vi "Periodic Tasks.vi"(8 "error in":errorcluster) -> ()   [LabVIEW 2018]
doc: "This VI runs in parallel to other tasks. It can contain as many user-defined periodic loops as you need. These can carry out PID or other sorts of timed response."
uses:
  <vilib>/Rock Robotics/WPI/ThirdParty/Phoenix-LabVIEW/Pigeon IMU/CTRE_PigeonIMU_CalibrationMode.ctl
  <vilib>/Rock Robotics/WPI/ThirdParty/Phoenix-LabVIEW/Pigeon IMU/CTRE_PigeonIMU_PigeonState.ctl
  DriveLoopEnum.ctl
  <vilib>/Rock Robotics/WPI/Utilities/WPI_GetSetVariantRefNum.vi
  <vilib>/Rock Robotics/WPI/ThirdParty/Phoenix-LabVIEW/Pigeon IMU/CTRE_PigeonIMU_GetTempStateUpTime.vi
  <vilib>/Rock Robotics/WPI/ThirdParty/Phoenix-LabVIEW/Pigeon IMU/CTRE_PigeonIMU_GetFusedHeading.vi
  <vilib>/Rock Robotics/WPI/ThirdParty/Phoenix-LabVIEW/Motor Controller/Get/CTRE_Phoenix_MotorController_GetVoltage.vi
  <vilib>/Rock Robotics/WPI/ThirdParty/Phoenix-LabVIEW/Motor Controller/Get/CTRE_Phoenix_MotorController_GetSelectedSensorData.vi
  <vilib>/Rock Robotics/WPI/ThirdParty/Phoenix-LabVIEW/Motor Controller/Get/CTRE_Phoenix_MotorController_GetClosedLoopData.vi
panel:
  out "Integral Accumulator":dbl
  out "Percent Power":T1(graph)
  out "Velocity":T2(graph)
  out "Error":cluster{"Closed-loop Error":i32, dbl, dbl}(graph)
  in  "D":dbl
  in  "I":dbl
  in  "P":dbl=1.0
  in  "Percent Max Speed":dbl=0.4
  in  "LowMaxSpeed":i32=7000
  out "Temp/State/UpTime":T5={"CurrentMode"=0, "LastCalError"=0, "CalBooting?"=FALSE, "PigeonState"=enum."Ready", "UpTime"=255, "Temp. (C)"=34.76953125, "Temp Compensation Event Count"=0, "No Motion Event Count"=0} {"CurrentMode" items=["BootTareGryoAccel"=0, "Temperature"=1, "Magnetometer12Pt"=2, "Magnetometer360"=3, "Accelerometer"=5]}
  out "Fused Heading":T6={"Heading"=373.0078125, "Valid?"=FALSE, "Fusing?"=FALSE}
  out "Right Position (Raw Sensor Units)":i32=1024961
  out "Left Position (Raw Sensor Units)":i32=868111
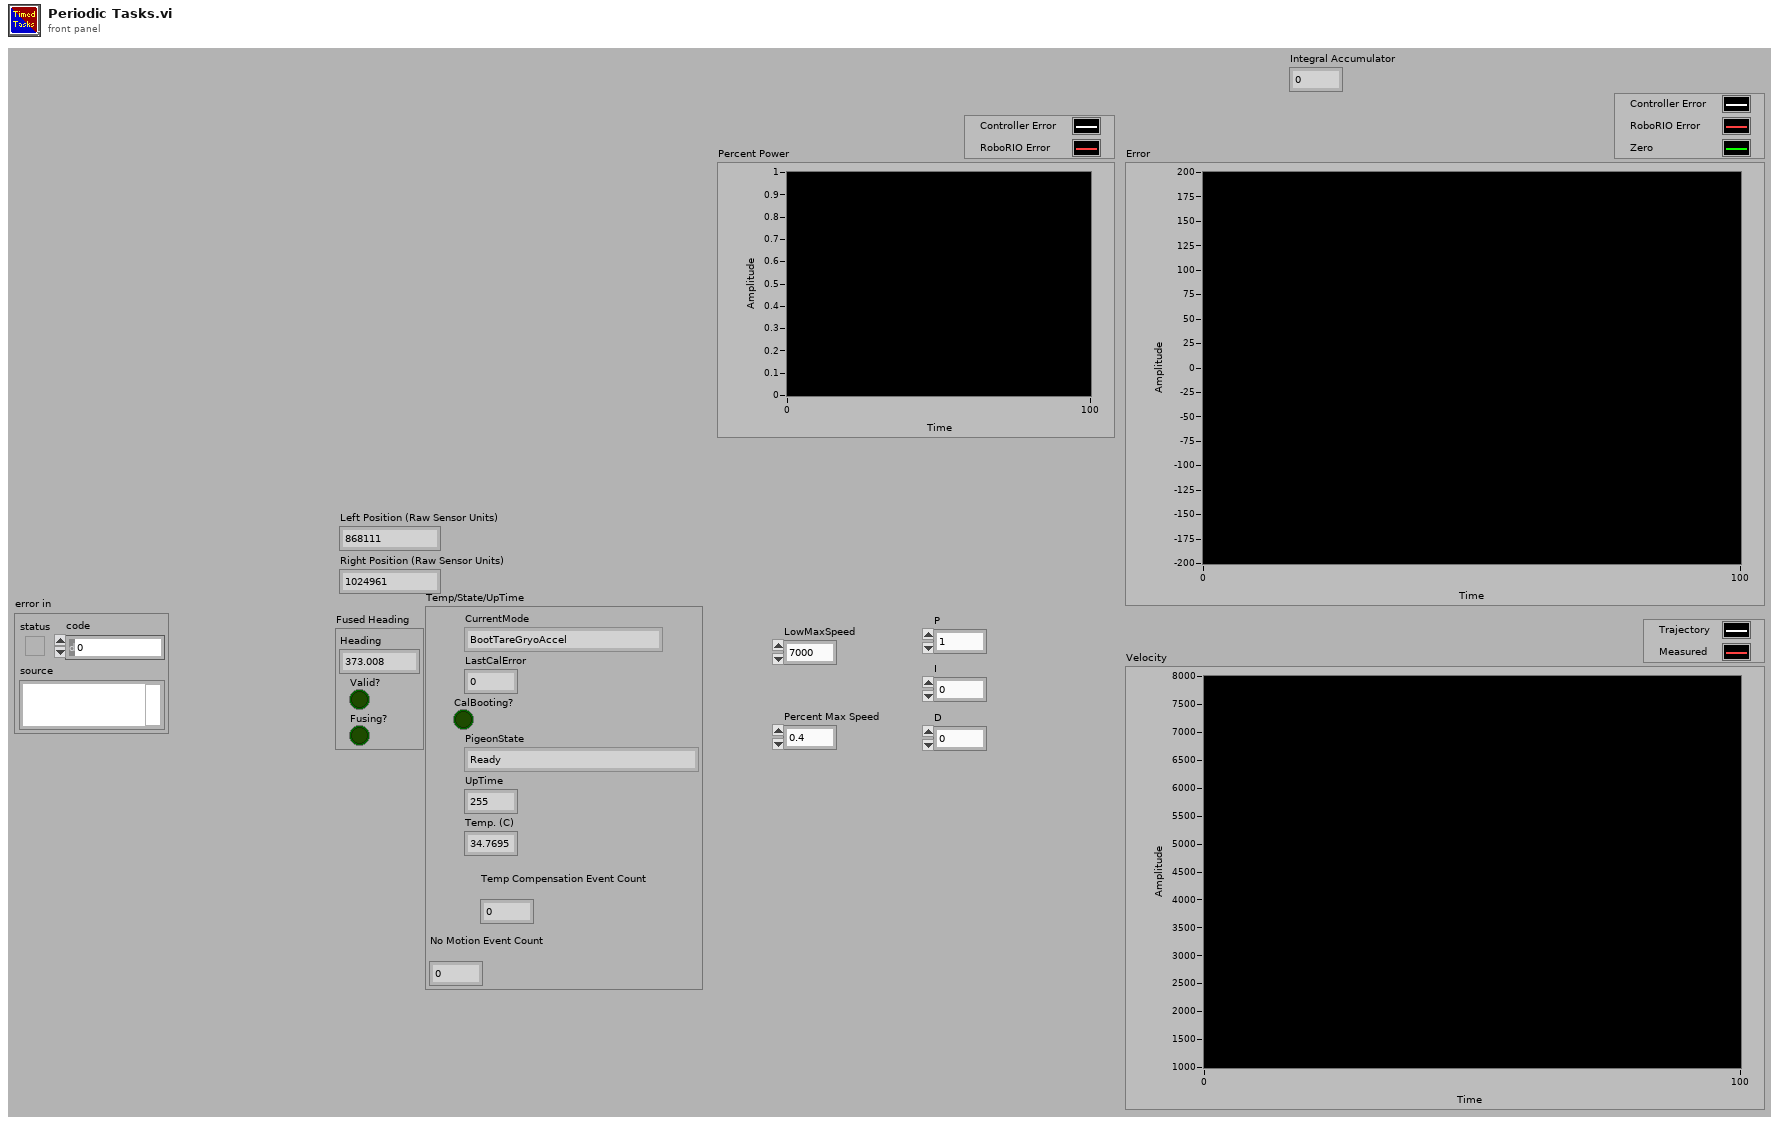
[diagram p1: front panel]
types:
  T1 = cluster{"Percent Output":dbl, "Percent Output":dbl}
  T2 = cluster{"Closed-loop Target":dbl, "Velocity (Raw Sensor Units per 100 ms)":i32}
  T3 = typedef "CTRE_PigeonIMU_CalibrationMode.ctl" = u16
  T4 = typedef "CTRE_PigeonIMU_PigeonState.ctl" = enum16{"NoComm", "Initializing", "Ready", "UserCalibration"}
  T5 = cluster{"CurrentMode":T3, "LastCalError":i32, "CalBooting?":bool, "PigeonState":T4, "UpTime":u32, "Temp. (C)":dbl, "Temp Compensation Event Count":u32, "No Motion Event Count":u32}
  T6 = cluster{"Heading":dbl, "Valid?":bool, "Fusing?":bool}
  T7 = typedef "CTRE_PigeonIMU_DeviceRef.ctl" = cluster{"DeviceStatus":errorcluster, "Device Number":u8, "Type":T8, "Device ID":u32, "Handle":u64, "UsageFrame":u32, "Library Path":path}
  T8 = typedef "CTRE_PigeonIMU_ConnectionType.ctl" = u32
  T9 = typedef "WPI_MotorControlDeviceRef.ctl" = cluster{"DeviceStatus":errorcluster, "Type":T10, "PWM":cluster{"PWM Channel":T11, "DeadBand":T12}, "CAN":cluster{"Device Number":u8, "SetOutput VI Ref":variant, "GetOutput VI Ref":variant, "Enable VI Ref":variant, "Disable VI Ref":variant, "Data":variant}, "Invert":bool, "DIO PWM":cluster{"PWM \"Enable\" Channel":T11, "DIOChannel":T13, "PWM Rate":dbl}}
  T10 = typedef "WPI_MotorControlType.ctl" = enum16{"PWM", "CAN", "DIO PWM"}
  T11 = typedef "FPGA_DIOPWMChannel.ctl" = enum8{"PWM 0", "PWM 1", "PWM 2", "PWM 3", "PWM 4", "PWM 5", "PWM 6", "PWM 7", "PWM 8", "PWM 9", "PWM MXP 0", "PWM MXP 1", "PWM MXP 2", "PWM MXP 3", "PWM MXP 4", "PWM MXP 5", "PWM MXP 6", "PWM MXP 7", "PWM MXP 8", "PWM MXP 9", "Invalid"}
  T12 = typedef "WPI_PWMDeadband.ctl" = cluster{"Name":string, "maxPositivePwm":i32, "minPositivePwm":i32, "centerPwm":i32, "maxNegativePwm":i32, "minNegativePwm":i32, "angularRange":u16}
  T13 = typedef "FPGA_DIOChannel.ctl" = enum8{"DIO 0", "DIO 1", "DIO 2", "DIO 3", "DIO 4", "DIO 5", "DIO 6", "DIO 7", "DIO 8", "DIO 9", "DIO MXP 0", "DIO MXP 1", "DIO MXP 2", "DIO MXP 3", "DIO MXP 4", "DIO MXP 5", "DIO MXP 6", "DIO MXP 7", "DIO MXP 8", "DIO MXP 9", "DIO MXP 10", "DIO MXP 11", "DIO MXP 12", "DIO MXP 13", "DIO MXP 14", "DIO MXP 15", "SPI Port CS1", "SPI Port CS2", "SPI Port CS3", "SPI Port MISO", "SPI Port MOSI", "Invalid"}
  T14 = typedef "WPI_JoystickDevRef.ctl" = cluster{"Device":T15}
  T15 = typedef "WPI_JoystickDeviceEnum.ctl" = enum16{"USB 0", "USB 1", "USB 2", "USB 3", "USB 4", "USB 5"}
  T16 = typedef "DriveLoopEnum.ctl" = enum16{"Manual", "Velocity Control", "Motion Magic"}
  T17 = cluster{dbl, "Velocity (Raw Sensor Units per 100 ms)":i32}
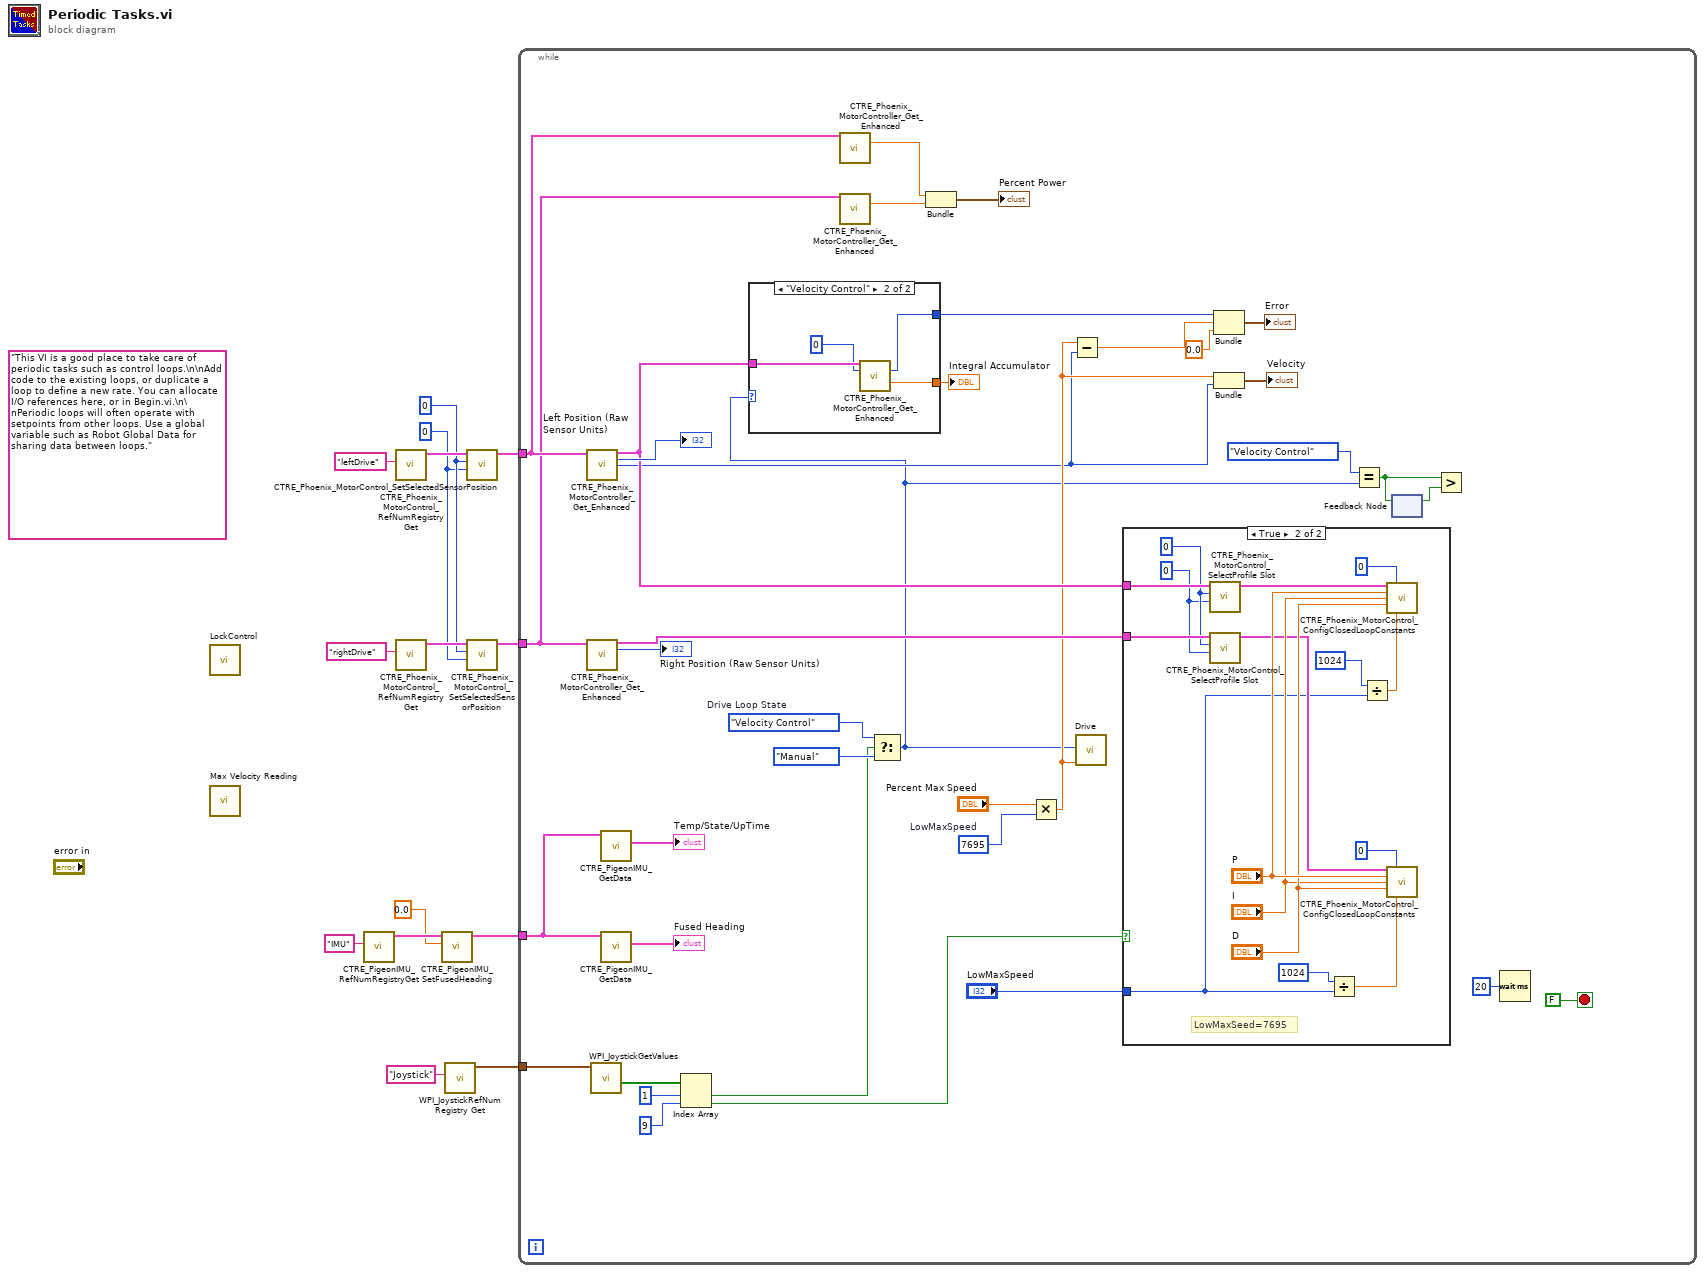
[diagram p0: block diagram]
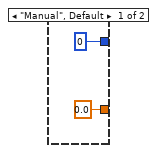
[diagram p2: hidden frame]
diagram:
  w7 = u32 0 ("pidLoopIdx")
  w8 = 0 ("New Sensor Position")
  (unwired) "This VI is a good place to take care of periodic tasks such as control loops.\n\nAdd code to the existing loops, or duplicate a loop to define a new rate. You can allocate I/O references here, or in Begin.vi.\n\nPeriodic loops will often operate with setpoints from other loops. Use a global variable such as Robot Global Data for sharing data between loops."
  n1 = call "LockControl.vi"() -> ()  [unwired: 12 in]
  n2 = call "Max Velocity Reading.vi"() -> ()  [unwired: 12 in]
  n3 = call <vilib>:"CTRE_PigeonIMU_RefNumRegistryGet.vi"("refnum name"="IMU") -> ("PigeonIMUDevRef"=w5:T7)  [unwired: 9 in, 1 out]
  n4 = call <vilib>:"CTRE_Phoenix_MotorControl_RefNumRegistryGet.vi"("refnum name"="leftDrive") -> ("PhoenixMotorControlDevRef"=w12:T9)  [unwired: 9 in, 1 out]
  n5 = call <vilib>:"CTRE_Phoenix_MotorControl_RefNumRegistryGet.vi"("refnum name"="rightDrive") -> ("PhoenixMotorControlDevRef"=w10:T9)  [unwired: 9 in, 1 out]
  n6 = call <vilib>:"CTRE_PigeonIMU_SetFusedHeading.vi"("Value"=0.0, "PigeonIMUDevRef 2"=w5) -> ("PigeonIMUDevRef"=w4:T7)  [unwired: 8 in, 1 out]
  n7 = call <vilib>:"WPI_JoystickRefNum Registry Get.vi"("refnum name"="Joystick") -> ("JoystickDevRef"=w1:T14)  [unwired: 9 in, 1 out]
  n8 = call <vilib>:"CTRE_Phoenix_MotorControl_SetSelectedSensorPosition.vi"("pidLoopIdx"=w7, "New Sensor Position"=w8, "PhoenixMotorControlDevRef"=w12) -> ("PhoenixMotorControlDevRef"=w11:T9)  [unwired: 7 in, 1 out]
  n9 = call <vilib>:"CTRE_Phoenix_MotorControl_SetSelectedSensorPosition.vi"("pidLoopIdx"=w7, "New Sensor Position"=w8, "PhoenixMotorControlDevRef"=w10) -> ("PhoenixMotorControlDevRef"=w9:T9)  [unwired: 7 in, 1 out]
  n10 = while {
    tunnel: w11 -> [w25]
    tunnel: w9 -> [w24]
    tunnel: w4 -> [w49]
    tunnel: w1 -> [w40]
    stop <- FALSE stop-if-true
    w42 = 7695  # LowMaxSpeed
    w44 = DriveLoopEnum."Velocity Control"  # Drive Loop State
    n11 = call-poly <vilib>:"CTRE_Phoenix_MotorController_Get_Enhanced.vi"("PhoenixMotorControlDevRef"=w25) -> ("PhoenixMotorControlDevRef"=w32:T9, "Position (Raw Sensor Units)"=→"Left Position (Raw Sensor Units)":i32, "Velocity (Raw Sensor Units per 100 ms)"=w26:i32)  [unwired: 11 in, 1 out]
    n12 = call-poly <vilib>:"CTRE_Phoenix_MotorController_Get_Enhanced.vi"("PhoenixMotorControlDevRef"=w24) -> ("PhoenixMotorControlDevRef"=w33:T9, "Position (Raw Sensor Units)"=→"Right Position (Raw Sensor Units)":i32)  [unwired: 11 in, 2 out]
    n13 = call <vilib>:"WPI_JoystickGetValues.vi"("JoystickDevRef"=w40) -> ("Buttons"=w39:bool[])  [unwired: 6 in, 4 out]
    n14 = call-poly <vilib>:"CTRE_PigeonIMU_GetData.vi"("PigeonIMUDevRef"=w49) -> ("Temp/State/UpTime"=→"Temp/State/UpTime":T5)  [unwired: 8 in, 2 out]
    n15 = call-poly <vilib>:"CTRE_PigeonIMU_GetData.vi"("PigeonIMUDevRef"=w49) -> ("Fused Heading"=→"Fused Heading":T6)  [unwired: 8 in, 2 out]
    n16 = Index Array(array=w39, index #1=1 ("index"), index #2=9 ("index")) -> (element #1=w36:bool, element #2=w38:bool)
    n17 = call-poly <vilib>:"CTRE_Phoenix_MotorController_Get_Enhanced.vi"("PhoenixMotorControlDevRef"=w25) -> ("Percent Output"=w23:dbl)  [unwired: 10 in, 4 out]
    n18 = call-poly <vilib>:"CTRE_Phoenix_MotorController_Get_Enhanced.vi"("PhoenixMotorControlDevRef"=w24) -> ("Percent Output"=w22:dbl)  [unwired: 10 in, 4 out]
    n19 = Select(t=w44, s=w36, f=DriveLoopEnum."Manual") -> (s? t:f=w18:T16)
    n20 = case shown="\"Velocity Control\"" w18 {
      tunnel: w32 -> [_ w57]
      tunnel: [0 ("Closed-loop Error") w55] -> w28
      tunnel: [0.0 ("Integral Accumulator") w54] -> w19
      frame "Manual", Default {
      }
      frame "Velocity Control" {
        n21 = call-poly <vilib>:"CTRE_Phoenix_MotorController_Get_Enhanced.vi"("PhoenixMotorControlDevRef"=w57, "pidLoopIdx"=0) -> ("Closed-loop Error"=w55:i32, "Integral Accumulator"=w54:dbl)  [unwired: 8 in, 4 out]
      }
    }
    "Integral Accumulator" <- w19
    n22 = Bundle("Percent Output"=w23, "Percent Output"=w22) -> (→"Percent Power":T1)  [unwired: 1 in]
    n23 = Multiply(x="Percent Max Speed", y=w42) -> (x*y=w27:dbl)
    n24 = Subtract(x=w27, y=w26) -> (x-y=w29:dbl)
    n25 = call "Drive.vi"("Velocity Setting"=w27, "Drive Loop State"=w18) -> ()  [unwired: 10 in]
    n26 = case shown="True" w38 {
      tunnel: "LowMaxSpeed" -> [_ w58]
      tunnel: w32 -> [_ w66]
      tunnel: w33 -> [_ w64]
      frame False {
      }
      frame True {
        w61 = 0 ("pidLoopIdx")
        w62 = 0 ("slotIdx")
        # "LowMaxSeed=7695"
        n27 = call <vilib>:"CTRE_Phoenix_MotorControl_SelectProfile Slot.vi"("pidLoopIdx"=w61, "slotIdx"=w62, "PhoenixMotorControlDevRef"=w66) -> ("PhoenixMotorControlDevRef"=w65:T9)  [unwired: 7 in, 1 out]
        n28 = call <vilib>:"CTRE_Phoenix_MotorControl_SelectProfile Slot.vi"("pidLoopIdx"=w61, "slotIdx"=w62, "PhoenixMotorControlDevRef"=w64) -> ("PhoenixMotorControlDevRef"=w63:T9)  [unwired: 7 in, 1 out]
        n29 = Divide(x=1024 ("y"), y=w58) -> (x/y=w73:dbl)
        n30 = Divide(x=1024 ("y"), y=w58) -> (x/y=w70:dbl)
        n31 = call <vilib>:"CTRE_Phoenix_MotorControl_ConfigClosedLoopConstants.vi"("PhoenixMotorControlDevRef"=w65, "slotIdx"=0, "P"="P", "I"="I", "D"="D", "F"=w70) -> ()  [unwired: 8 in, 2 out]
        n32 = call <vilib>:"CTRE_Phoenix_MotorControl_ConfigClosedLoopConstants.vi"("PhoenixMotorControlDevRef"=w63, "slotIdx"=0, "P"="P", "I"="I", "D"="D", "F"=w73) -> ()  [unwired: 8 in, 2 out]
      }
    }
    n33 = Bundle("Closed-loop Error"=w28, w29, 0.0) -> (→"Error":cluster{"Closed-loop Error":i32, dbl, dbl})  [unwired: 1 in]
    n34 = Bundle(w27, "Velocity (Raw Sensor Units per 100 ms)"=w26) -> (→"Velocity":T17)  [unwired: 1 in]
    n35 = Equal?(x=DriveLoopEnum."Velocity Control", y=w18) -> (x = y?=w15:bool)
    n36 = feedback-in #1(w15) -> ()
    n37 = feedback #1() -> (w16:bool)  [unwired: 1 in]
    n38 = Greater?(x=w15, y=w16) -> ()  [unwired: 1 out]
    n39 = Wait (ms)(milliseconds to wait=u32 20) -> ()  [unwired: 1 out]
  }
